vi "hw1-1 topVI.vi"() -> ()   [LabVIEW 2014]
panel:
  out "min":dbl
  out "max":dbl
  out "avg val.":dbl
  out "hw1-1-4 plot":T1(graph)
  out "hw1-1-3 temp val from thermometer.vi":dbl(graph)
  in  "degC/degF":bool
  in  "Summer/Winter":enum16{"Summer", "Winter"}(ring)
  in  "stop":bool
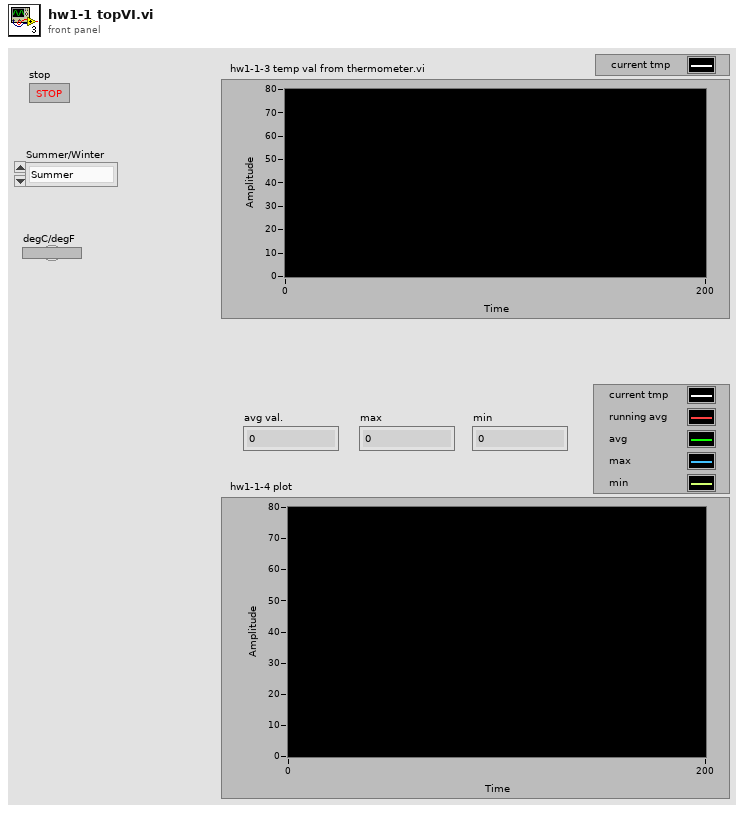
[diagram p1: front panel]
types:
  T1 = cluster{"random degC":dbl, dbl, dbl, "random degC":dbl, "random degC":dbl}
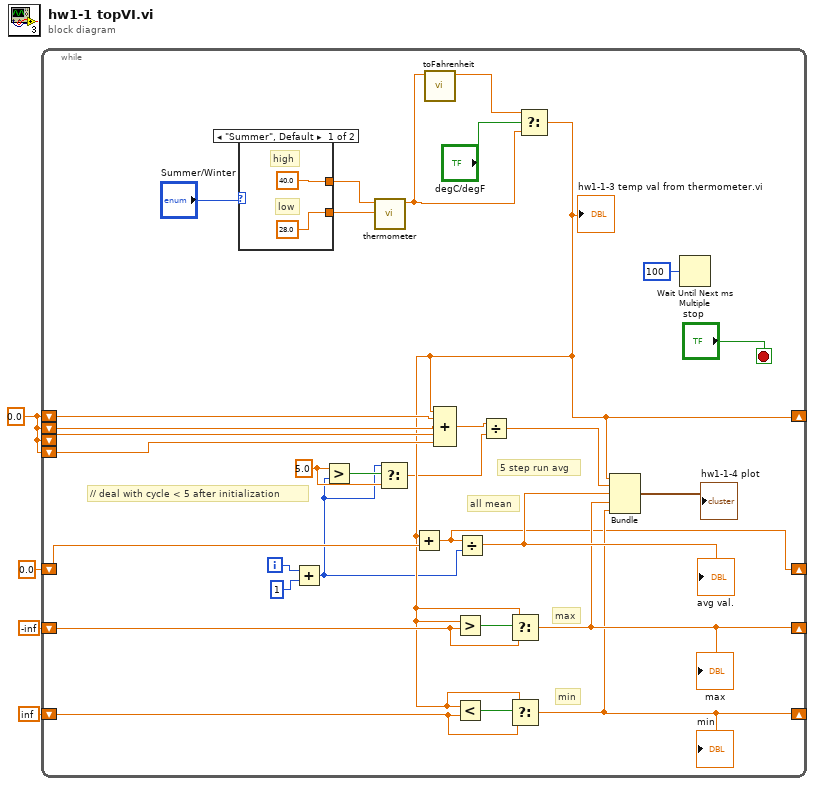
[diagram p0: block diagram]
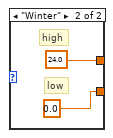
[diagram p2: hidden frame]
diagram:
  w4 = 0.0 ("random degC")
  n1 = while {
    shift-right: [w12] -> _
    shift-left: w4 -> [w27]
    shift-left: w4 -> [w26]
    shift-left: w4 -> [w25]
    shift-left: w4 -> [w24]
    shift-right: [w9] -> _
    shift-left: 0.0 ("random degC") -> [w16]
    shift-right: [w14] -> _
    shift-left: -inf ("random degC") -> [w15]
    shift-right: [w10] -> _
    shift-left: inf ("random degC") -> [w11]
    i -> [w20]
    stop <- "stop" stop-if-true
    w6 = 5.0 ("x")
    # "// deal with cycle < 5 after initialization"
    # "min"
    # "max"
    # "all mean"
    # "5 step run avg"
    n2 = case shown="\"Summer\", Default" "Summer/Winter" {
      tunnel: [40.0 24.0] -> w33
      tunnel: [28.0 0.0] -> w32
      frame "Summer", Default {
        # "low"
        # "high"
      }
      frame "Winter" {
        # "low"
        # "high"
      }
    }
    n3 = Add(x=w20, y=1) -> (x+y=w5:i32)
    n4 = Greater?(x=w6, y=w5) -> (0:w8:bool)
    n5 = call "thermometer.vi"("lower bound value"=w32, "upper bound value"=w33) -> ("random degC"=w28:dbl)  [unwired: 9 in]
    n6 = Select(t=w5, s=w8, f=w6) -> (s? t:f=w7:dbl)
    n7 = call "toFahrenheit.vi"("degC"=w28) -> ("degF"=w29:dbl)  [unwired: 10 in]
    n8 = Select(t=w29, s="degC/degF", f=w28) -> (s? t:f=w12:dbl)
    "hw1-1-3 temp val from thermometer.vi" <- w12
    n9 = Add(x=w12, y=w16) -> (x+y=w9:dbl)
    n10 = Compound Arithmetic op=ADD(w12, w27, w26, w25, w24) -> (w23:dbl)
    n11 = Greater?(x=w12, y=w15) -> (0:w17:bool)
    n12 = Less?(x=w12, y=w11) -> (x < y?=w13:bool)
    n13 = Divide(x=w9, y=w5) -> (x/y=w18:dbl)
    "avg val." <- w18
    n14 = Divide(x=w23, y=w7) -> (x/y=w21:dbl)
    n15 = Select(t=w12, s=w17, f=w15) -> (s? t:f=w14:dbl)
    "max" <- w14
    n16 = Select(t=w12, s=w13, f=w11) -> (s? t:f=w10:dbl)
    "min" <- w10
    n17 = Bundle("random degC"=w12, w21, w18, "random degC"=w14, "random degC"=w10) -> (→"hw1-1-4 plot":T1)  [unwired: 1 in]
    n18 = Wait Until Next ms Multiple(millisecond multiple=u32 100) -> ()  [unwired: 1 out]
  }
